vi "Vision Processing.vi"() -> ()   [LabVIEW 2011]
uses:
  signals/Signal.ctl
  <vilib>/Rock Robotics/WPI/Camera/WPI_CameraImageSize.ctl
  <vilib>/vision/NI_Vision_Development_Module.lvlib
panel:
  out "Delta-T":u32
  in  "Range":cluster{"Lower value":sgl, "Upper value":sgl}={"Lower value"=214.34782, "Upper value"=255.0} {"Lower value" scale=0.0..255.0; "Upper value" scale=0.0..255.0}
  in  "View":bool
  in  "Area Size Limit":i32=444
  in  "Particle Count Limit":i32=8
  in  "Score Limits":T1={"Rect Coverage"=76.0, "Aspect Ratio"=0.0, "X Edge Strength"=40.0, "Y Edge Strength"=50.0}
  in  "View":bool
  out "Processed Image":T2(plugin-control)
  out "Original Image":T2(plugin-control)
  # "Instructions:\nProcessing the reflective tape that is illuminated by a ring light can be based\non color or light intensity.\nParticles within the image are scored by rectangle coverage, aspect ratio, and\nfor being hollow with a bold edge. A particle is considered a target if all scores\nare above the score limits. Particles can be annotated -- surrounded by\na rectangle and scores drawn to the left .\nTo control the number of particles being scored, use the count limit and the size\nlimit."
  # "To debug, Enable using the View button.\nFor color processing, you can click in the image to select the color for processing."
  # "Enable by clicking the View button.\nGreen scores are above the limit, orange are below. Inner/outer rect\nindicates all passed."
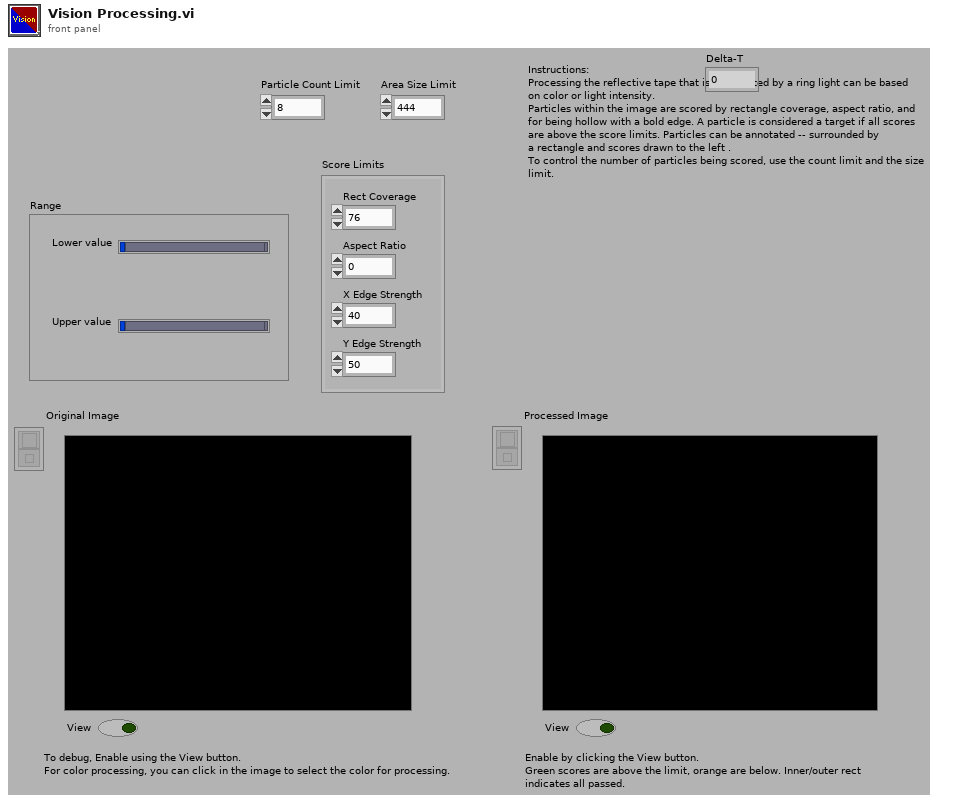
[diagram p1: front panel]
types:
  T1 = cluster{"Rect Coverage":dbl, "Aspect Ratio":dbl, "X Edge Strength":dbl, "Y Edge Strength":dbl}
  T2 = typedef "IMAQ Image.ctl" = refnum<image>
  T3 = typedef "Image Type" = u32
  T4 = typedef "WPI_CameraDevRef.ctl" = cluster{"Camera Address":string, "CameraStatus":errorcluster, "Acquire Image Notifier":refnum<notifier>}
  T5 = typedef "Signal.ctl" = enum16{"SIGFIRE", "SIGSTOPSCRIPT", "SIGSTARTGUN", "SIGSTOPGUN", "SIGDISABLED", "SIGENABLED", "SIGUDPTIMEOUT", "SIGNEWVISION_REMOTE", "SIGNEWVISION_LOCAL", "SIGSHOTFIRED", "SIGDOTRACK", "SIGDONTTRACK"}
  T6 = typedef "WPI_CameraImageSize.ctl" = enum16{"640x480", "320x240", "160x120"}
  T7 = enum32{"AutoM", "Close", "Dilate", "Erode", "Gradient", "Gradient out", "Gradient in", "Hit miss", "Open", "PClose", "POpen", "Thick", "Thin"}
  T8 = enum16{"Get Latest Data", "Get Local Data", "Get Remote Data", "Set Local Data", "Set Remote Data"}
  T9 = cluster{cluster{"Left":dbl, "Top":dbl, "Right":dbl, "Bottom":dbl}, cluster{"Score":dbl, "Score":dbl, "X Score":dbl, "Y Score":dbl}, "Clipped Edge":cluster{"Left":bool, "Top":bool, "Right":bool, "Bottom":bool}}[]
  T10 = typedef "Camera State.ctl" = enum16{"No Targets", "Low Confidence", "Medium Confidence", "High Confidence", "Camera Error"}
  T11 = cluster{"X Position":dbl, "Distance":dbl, "Camera State":T10}
  T12 = typedef "Diamond Target Output.ctl" = cluster{"Position":cluster{"X":dbl, "Y":dbl, "Distance":dbl}, "Est. Position":T13, "Target Confidence":T14}
  T13 = typedef "Rectangle Position.ctl" = enum16{"Unknown", "Top", "Right", "Left", "Bottom"}
  T14 = typedef "Target Confidence.ctl" = enum16{"Good", "Good-Clipped Y", "Marginal-Clipped X"}
  T15 = typedef "Line.ctl" = cluster{"First Point":cluster{"X":dbl, "Y":dbl, "Index":dbl}, "Second Point":cluster{"X":dbl, "Y":dbl, "Index":dbl}, "theta":dbl, "Direction":T16, "Line Confidence":T17}
  T16 = typedef "Direction.ctl" = enum16{"Rt", "Rt-Up", "Up", "Lt-Up", "Lt", "Lt-Dn", "Dn", "Rt-Dn", "Unknown"}
  T17 = typedef "Line Confidence.ctl" = enum16{"Good", "Bad"}
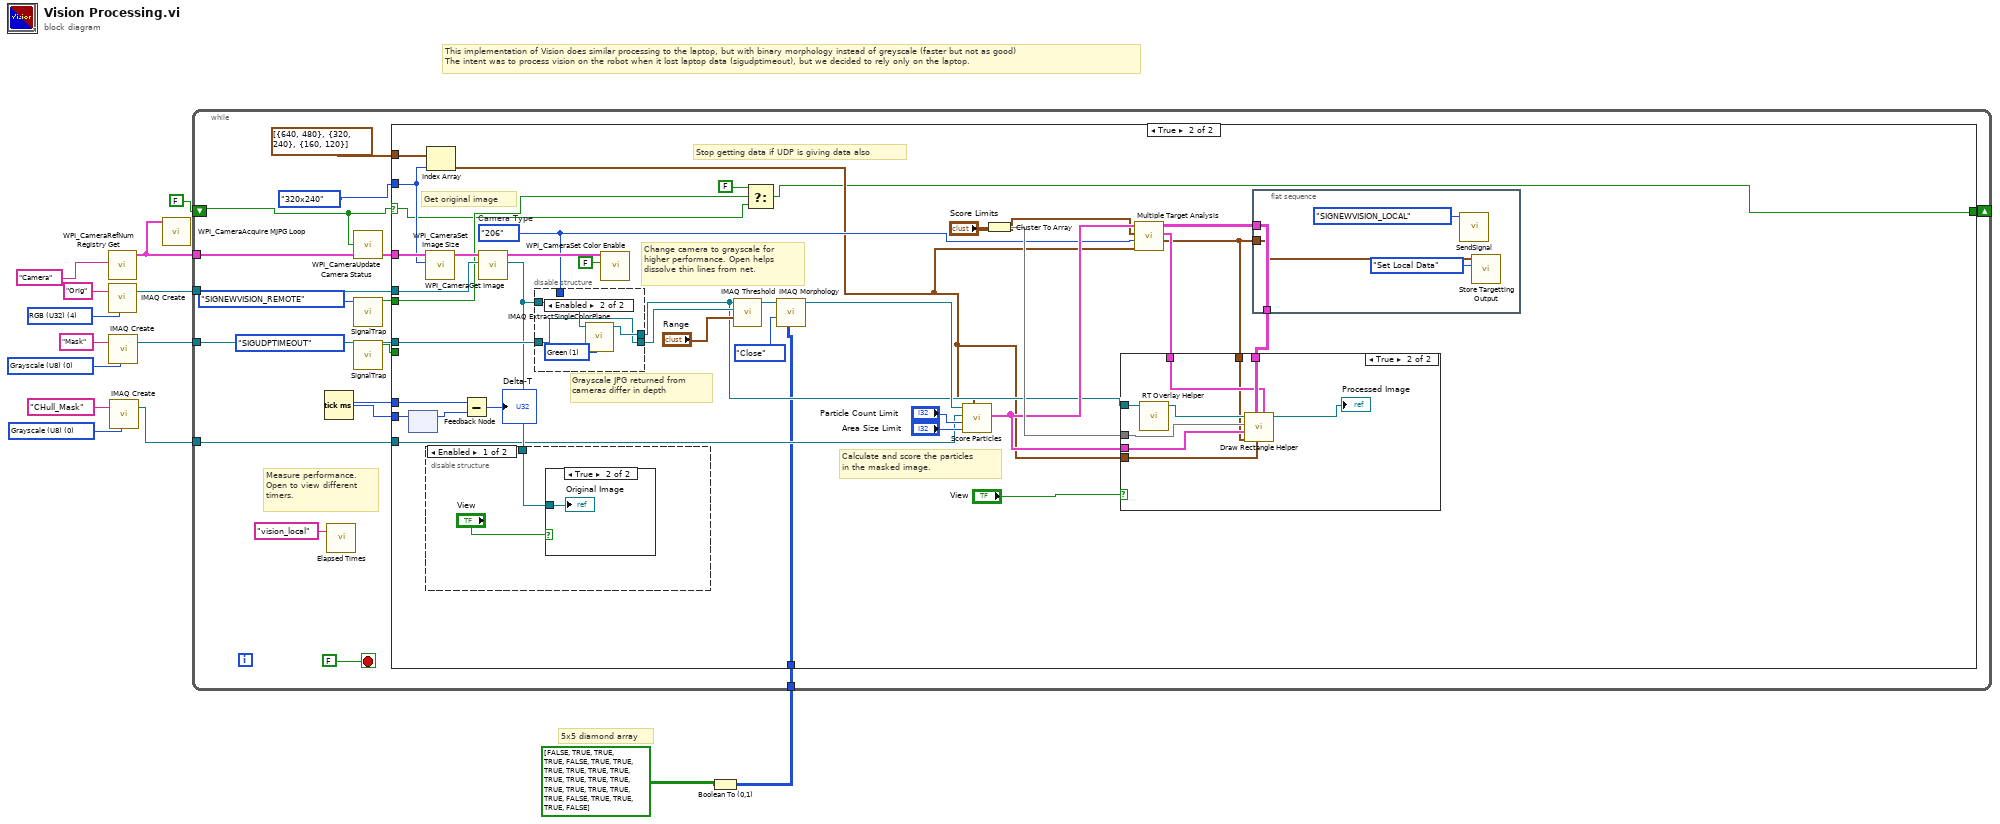
[diagram p0: block diagram]
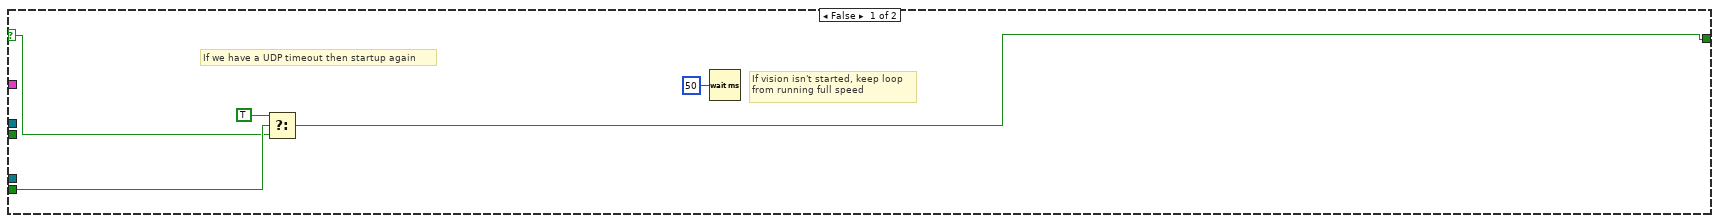
[diagram p2: hidden frame]
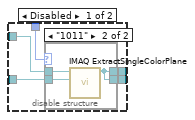
[diagram p3: hidden frame]
diagram:
  w6 = T3 0 items=["Grayscale (U8)", "Grayscale (I16)", "Grayscale (SGL)", "Complex (CSG)", "RGB (U32)", "HSL (U32)", "RGB (U64)", "Grayscale (U16)"] ("Image Type")
  w9 = T3 0 items=["Grayscale (U8)", "Grayscale (I16)", "Grayscale (SGL)", "Complex (CSG)", "RGB (U32)", "HSL (U32)", "RGB (U64)", "Grayscale (U16)"] ("Image Type")
  w13 = T3 4 items=["Grayscale (U8)", "Grayscale (I16)", "Grayscale (SGL)", "Complex (CSG)", "RGB (U32)", "HSL (U32)", "RGB (U64)", "Grayscale (U16)"] ("Image Type")
  # "This implementation of Vision does similar processing to the laptop, but with binary morphology instead of greyscale (faster but not as good)\nThe intent was to process vision on the robot when it lost laptop data (sigudptimeout), but we decided to rely only on the laptop."
  # "5x5 diamond array"
  n1 = call <vilib>:"WPI_CameraRefNum Registry Get.vi"("refnum name"="Camera" ("Camera Name")) -> ("CameraDevRef"=w10:T4)  [unwired: 9 in, 1 out]
  n2 = call "IMAQ Create"("Image Name"="Orig", "Image Type"=w13) -> ("New Image"=w12:T2)  [unwired: 2 in, 2 out]
  n3 = call "IMAQ Create"("Image Name"="Mask", "Image Type"=w9) -> ("New Image"=w7:T2)  [unwired: 2 in, 2 out]
  n4 = call "IMAQ Create"("Image Name"="CHull_Mask", "Image Type"=w6) -> ("New Image"=w4:T2)  [unwired: 2 in, 2 out]
  n5 = call <vilib>:"WPI_CameraAcquire MJPG Loop.vi"("CameraDevRef"=w10) -> ()  [unwired: 11 in]
  n6 = Boolean To (0,1)(Boolean=bool[][] [[FALSE, TRUE, TRUE, TRUE, FALSE], [TRUE, TRUE, TRUE, TRUE, TRUE], [TRUE, TRUE, TRUE, TRUE, TRUE], [TRUE, TRUE, TRUE, TRUE, TRUE], [FALSE, TRUE, TRUE, TRUE, FALSE]]) -> (0, 1=w1:i16[][])
  n7 = while {
    tunnel: w12 -> [w29]
    tunnel: w10 -> [w28]
    tunnel: w7 -> [w25]
    tunnel: w4 -> [w21]
    shift-right: [w17] -> _
    shift-left: FALSE -> [w20]
    tunnel: w1 -> [w15]
    stop <- FALSE stop-if-true
    (unwired) Signal."SIGUDPTIMEOUT" ("Signal")
    # "Measure performance.\nOpen to view different\ntimers."
    n8 = Tick Count (ms)() -> (millisecond timer value=w22:u32)
    n9 = call "Elapsed Times.vi"("Call Name"="vision_local") -> ()  [unwired: 2 in, 1 out]
    n10 = call <vilib>:"WPI_CameraUpdate Camera Status.vi"("CameraDevRef In"=w28, "Enable Vision"=w20) -> ("CameraDevRef Out"=w27:T4)  [unwired: 3 in]
    n11 = call "SignalTrap.vi"("Signal"=Signal."SIGNEWVISION_REMOTE") -> ("Trapped Signal"=w18:bool)  [unwired: 10 in]
    n12 = call "SignalTrap.vi"() -> ("Trapped Signal"=w16:bool)  [unwired: 11 in]
    n13 = case shown="True" w20 {
      selector: w20 -> [w33 w39]
      tunnel: w29 -> [_ w68]
      tunnel: w27 -> [_ w65]
      tunnel: WPI_CameraImageSize."320x240" ("Image Size") -> [_ w63]
      tunnel: w25 -> [_ w61]
      tunnel: cluster{i32, i32}[] [{640, 480}, {320, 240}, {160, 120}] -> [_ w62]
      tunnel: w22 -> [_ w54]
      tunnel: w22 -> [_ w53]
      tunnel: w21 -> [_ w46]
      tunnel: w18 -> [_ w40]
      tunnel: [w31 w37] -> w17
      tunnel: w16 -> [w34 _]
      tunnel: w15 -> [_ w36]
      frame False {
        # "If we have a UDP timeout then startup again"
        # "If vision isn't started, keep loop\nfrom running full speed"
        n14 = Select(t=TRUE, s=w34, f=w33) -> (s? t:f=w31:bool)
        n15 = Wait (ms)(milliseconds to wait=u32 50) -> ()  [unwired: 1 out]
      }
      frame True {
        w48 = enum16{"206", "1011"}."206"  # Camera Type
        # "Stop getting data if UDP is giving data also"
        # "Grayscale JPG returned from\ncameras differ in depth"
        # "Change camera to grayscale for\nhigher performance. Open helps\ndissolve thin lines from net."
        # "Calculate and score the particles\nin the masked image."
        # "Get original image"
        n16 = feedback-in #1(w53) -> ()
        n17 = feedback #1() -> (w52:u32)  [unwired: 1 in]
        n18 = call <vilib>:"WPI_CameraSet Image Size.vi"("Image Size"=w63, "CameraDevRef"=w65) -> ("CameraDevRef Out"=w66:T4)  [unwired: 8 in, 1 out]
        n19 = Index Array(array=w62, index=w63) -> (element=w44:cluster{i32, i32})
        n20 = Subtract(x=w54, y=w52) -> (x-y=→"Delta-T":u32)
        n21 = call <vilib>:"WPI_CameraGet Image.vi"("Image"=w68, "CameraDevRef"=w66) -> ("Image Out"=w60:T2, "CameraDevRef Out"=w67:T4)  [unwired: 7 in, 1 out]
        n22 = disable-structure shown="Enabled" {
          disable-tunnel: w60 -> [w91 _]
          frame Enabled {
            n23 = case shown="True" "View" {
              tunnel: w91 -> [_ w93]
              frame False {
              }
              frame True {
                "Original Image" <- w93
              }
            }
          }
          frame Disabled {
          }
        }
        n24 = disable-structure shown="Enabled" {
          disable-tunnel: w61 -> [w81 w87]
          disable-tunnel: w60 -> [w80 w90]
          disable-tunnel: [w79 w87] -> w55
          disable-tunnel: w48 -> [w78 _]
          disable-tunnel: [w77 w88] -> w45
          frame Disabled {
            n25 = case shown="\"1011\"" w78 {
              tunnel: w80 -> [w83 w86]
              tunnel: w81 -> [w82 w85]
              tunnel: [w83 w84] -> w77
              tunnel: [w82 w84] -> w79
              frame "206", Default {
              }
              frame "1011" {
                n26 = call "IMAQ ExtractSingleColorPlane"("Image Dst"=w85, "Image Src"=w86) -> ("Image Dst Out"=w84:T2)  [unwired: 8 in, 1 out]
              }
            }
          }
          frame Enabled {
            w89 = 1 items=["Red", "Green", "Blue", "Hue", "Saturation", "Luminance", "Value", "Intensity"] ("Color Plane")
            n27 = call "IMAQ ExtractSingleColorPlane"("Color Plane"=w89, "Image Src"=w90) -> ("Image Dst Out"=w88:T2)  [unwired: 8 in, 1 out]
          }
        }
        n28 = call <vilib>:"WPI_CameraSet Color Enable.vi"("Color Enabled"=FALSE, "CameraDevRef"=w67) -> ()  [unwired: 8 in, 2 out]
        n29 = call "IMAQ Threshold"("Range"="Range", "Image Dst"=w55, "Image Src"=w45) -> ("Image Dst Out"=w57:T2)  [unwired: 3 in, 5 out]
        n30 = Select(t=FALSE, s=w40, f=w39) -> (s? t:f=w37:bool)
        n31 = call "IMAQ Morphology"("Structuring Element"=w36, "Operation"=T7."Close", "Image Src"=w57) -> ("Image Dst Out"=w64:T2)  [unwired: 7 in, 1 out]
        n32 = call "Score Particles.vi"("Image Size"=w44, "Area Size Limit"="Area Size Limit", "Particle Count Limit"="Particle Count Limit", "Image Dst"=w46, "Image Refnum in"=w64) -> ("Targets"=w50:T9)  [unwired: 5 in, 1 out]
        n33 = Cluster To Array(cluster="Score Limits") -> (array=w71:dbl[])
        n34 = call "Multiple Target Analysis.vi"("Image Size"=w44, "Camera Type"=w48, "Score Limits"="Score Limits", "Targets"=w50) -> ("Targetting Output"=w41:T11, "Diamond Targets"=w47:T12[], "Lines"=w42:T15[][])  [unwired: 5 in]
        n35 = case shown="True" "View" {
          tunnel: w45 -> [_ w99]
          tunnel: w50 -> [_ w101]
          tunnel: w71 -> [_ w100]
          tunnel: w43 -> [_ w97]
          tunnel: w47 -> [_ w96]
          tunnel: w41 -> [_ w95]
          tunnel: w44 -> [_ w94]
          frame False {
          }
          frame True {
            n36 = call "RT Overlay Helper.vi"("Refnum in"=w99) -> ("Refnum out"=w102:T2)  [unwired: 10 in]
            n37 = call "Draw Rectangle Helper.vi"("Diamond Targets"=w96, "Image Size"=w94, "Lines"=w97, "Targetting Output"=w95, "Targets"=w101, "Score Limits"=w100, "Refnum in"=w102) -> ("Refnum out"=→"Processed Image":T2)  [unwired: 4 in]
          }
        }
        n38 = flat-sequence {
          tunnel: [w76] -> w43
          tunnel: w42 -> [w76]
          tunnel: w41 -> [w74]
          frame #0 {
            n39 = call "SendSignal.vi"("Signal"=Signal."SIGNEWVISION_LOCAL") -> ()  [unwired: 11 in]
            n40 = call "Store Targetting Output.vi"("mode"=T8."Set Local Data", "Targetting Input"=w74) -> ()  [unwired: 9 in, 1 out]
          }
        }
      }
    }
  }
